vi "WriteRegister.vi"(5 "Registers Info":map{T1, T2}(c390), 7 "Device Address":u8, 8 "error in (no error)":errorcluster, 9 "Register Name":T1=enum."Frame Rate", 10 "DATA":u8[](array[numeric]), 11 "II2COUSB":refnum<class "II2COUSB.lvclass">) -> (0 "error out":errorcluster, 3 "II2COUSB out":refnum<class "II2COUSB.lvclass">)   [LabVIEW 2020, in "CameraI2COUSB.lvlib" / "CameraI2COUSB.lvclass"]
uses:
  CameraI2COUSB.lvclass
  TypeDef/RegisterName.ctl
  TypeDef/RegisterInfo.ctl
  CameraDriver/II2COUSB/II2COUSB/II2COUSB.lvclass
  CameraDriver/II2COUSB/TypeDef/I2CFlags.ctl
  CameraI2COUSB.lvclass/CameraI2COUSB.ctl
  CameraDriver/II2COUSB/TypeDef/II2COUSB_typedef.lvlib
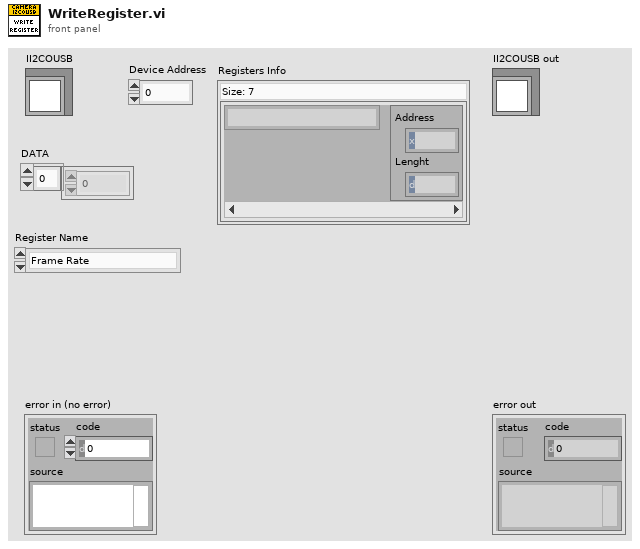
[diagram p1: front panel]
types:
  T1 = typedef "CameraI2COUSB.lvlib/CameraI2COUSB.lvclass/RegisterName.ctl" = enum16{"Clock Rate", "Frame Rate", "Image Type", "Resolution", "Snap", "Start Streaming", "Stop Streaming"}
  T2 = typedef "CameraI2COUSB.lvlib/CameraI2COUSB.lvclass/RegisterInfo.ctl" = cluster{"Address":u16, "Lenght":u32}
  T3 = typedef "II2COUSB_typedef.lvlib/I2CFlags.ctl" = u8
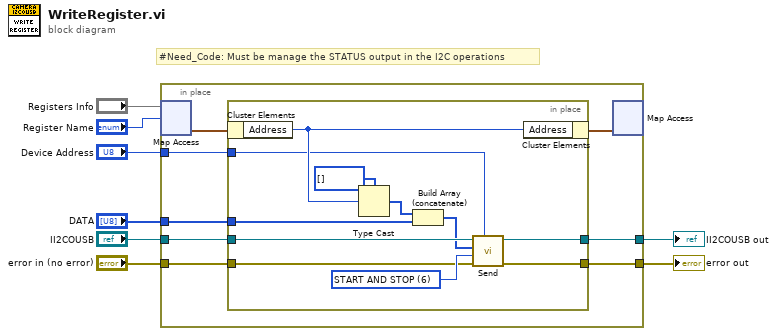
[diagram p0: block diagram]
diagram:
  # "#Need_Code: Must be manage the STATUS output in the I2C operations"
  n1 = in-place {
    in-place-border: "II2COUSB" -> [w15]
    in-place-border: "error in (no error)" -> [w14]
    in-place-border: [w10] -> w3
    in-place-border: "Device Address" -> [w13]
    in-place-border: "DATA" -> [w11]
    in-place-border: [w9] -> w1
    n2 = in-place-map #1("Registers Info", "Register Name") -> (w16:T2)  [unwired: 1 in, 1 out]
    n3 = in-place {
      in-place-border: w15 -> [w23]
      in-place-border: w14 -> [w24]
      in-place-border: w13 -> [w22]
      in-place-border: w11 -> [w20]
      in-place-border: [w18] -> w10
      in-place-border: [w17] -> w9
      w26 = T3 6 items=["None"=0, "START"=2, "REPEATED START"=3, "STOP"=4, "START AND STOP"=6] ("eI2Cflags")
      n4 = in-place-cluster #2(w16) -> ("Address"=w25:u16)
      n5 = Type Cast(type=u8[] [], x=w25) -> (*(type *) &x=w21:u8[])
      n6 = Build Array (concatenate)(w21, w20) -> (w19:u8[])
      n7 = call-dynamic "Send.vi"("Device Address"=w22, "error in (no error)"=w24, "eI2Cflags"=w26, "Buffer"=w19, "II2COUSB in"=w23) -> ("error out"=w18:errorcluster, "II2COUSB out"=w17:refnum<class "II2COUSB.lvclass">)  [unwired: 3 in, 2 out]
      n8 = in-place-cluster #2("Address"=w25) -> (w12:T2)
    }
    n9 = in-place-map #1(w12) -> ()  [unwired: 1 in, 3 out]
  }
  "error out" <- w3
  "II2COUSB out" <- w1
